vi "Get Cell Data.vi"(8 "error in (no error)":errorcluster, 9 "Row Index":i32, 10 "Header":string, 11 "SLL Table in":refnum<class "SLL Table.lvclass">) -> (0 "error out":errorcluster, 1 "Header Present?":bool, 2 "Cell Data":string, 3 "SLL Table out":refnum<class "SLL Table.lvclass">)   [LabVIEW 2016, in "SLL Table.lvclass"]
doc: "Returns the cell data for the specified column and row index."
uses:
  SLL Table.lvclass
  SLL Table.lvclass/SLL Table.ctl
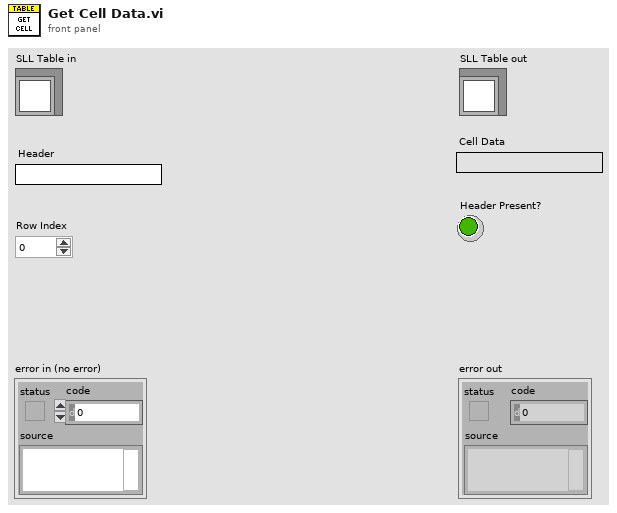
[diagram p1: front panel]
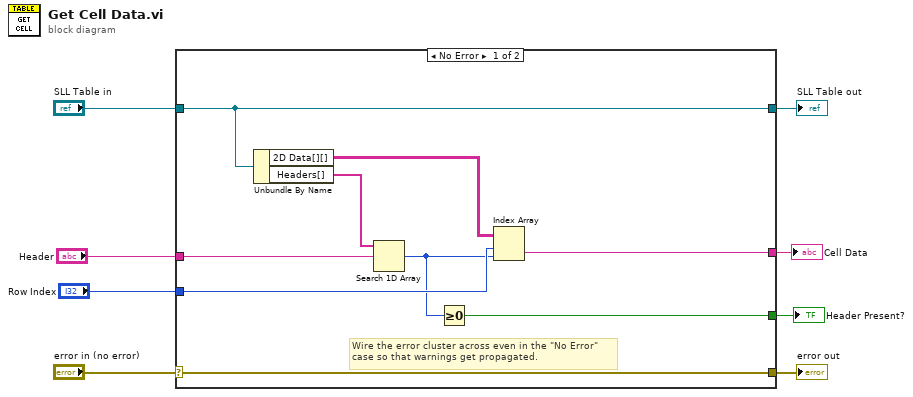
[diagram p0: block diagram]
diagram:
  n1 = case shown="No Error" "error in (no error)" {
    selector: "error in (no error)" -> [w17 w19]
    tunnel: [w17 w19] -> w7
    tunnel: [w16 w18] -> w5
    tunnel: "SLL Table in" -> [w16 w18]
    tunnel: "Header" -> [w14 _]
    tunnel: [w13 _] -> w2
    tunnel: "Row Index" -> [w12 _]
    tunnel: [w10 _] -> w1
    frame No Error {
      # "Wire the error cluster across even in the \"No Error\"\ncase so that warnings get propagated."
      n2 = Unbundle By Name(w16) -> ("2D Data[][]"=w9:string[][], "Headers[]"=w15:string[])
      n3 = Search 1D Array(1D array=w15, element=w14) -> (index of element=w11:i32)  [unwired: 1 in]
      n4 = Greater Or Equal To 0?(x=w11) -> (x >= 0?=w10:bool)
      n5 = Index Array(array=w9, index (row)=w12, index (col)=w11) -> (element=w13:string)
    }
    frame Error {
    }
  }
  "error out" <- w7
  "SLL Table out" <- w5
  "Cell Data" <- w2
  "Header Present?" <- w1
